vi "three_button.vi"(7 "callee":refnum<vi>, 8 "error in (no error)":errorcluster, 11 "configuration":T2={"dialog_text"="", "boolean_text_1"="", "boolean_text_2"="", "boolean_text_3"="", "inner_color"=16711680, "outer_color"=6618880, "wait_s"=nan, "error_status"=FALSE, "error_source"="", "error_details"="", "string []"=[], "custom_entry"=FALSE}) -> (0 "error out":errorcluster, 3 "dialog_selection":T1)   [LabVIEW 2015, in "lv-dialog-interfaces.lvlib"]
uses:
  lv-dialog-interfaces.lvlib
  lv-dialog/api/v1/public/_controls/configuration.ctl
  lv-dialog/api/v1/public/_controls/dialog_selection.ctl
  _controls/dialog_type.ctl
  _controls/hmi_references.ctl
  <vilib>/event_ctls.llb/eventvkey.ctl
  lv-dialog/api/v1/v1.lvlib
panel:
  out "dialog":string
  in  "button_1":bool
  in  "button_2":bool
  in  "button_3":bool
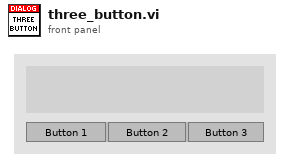
[diagram p1: front panel]
types:
  T1 = typedef "lv-dialog.lvlib/v1.lvlib/dialog_selection.ctl" = enum16{"null", "panel_closed", "button_1", "button_2", "button_3", "cancelled"}
  T2 = typedef "lv-dialog.lvlib/v1.lvlib/configuration.ctl" = cluster{"dialog_text":string, "boolean_text_1":string, "boolean_text_2":string, "boolean_text_3":string, "inner_color":u32, "outer_color":u32, "wait_s":dbl, "error_status":bool, "error_source":string, "error_details":string, "string []":string[], "custom_entry":bool}
  T3 = typedef "lv-dialog-interfaces.lvlib/dialog_type.ctl" = enum16{"null", "one_button", "two_button", "three_button", "confirmation", "busy_wait", "error", "busy_wait_embed", "combo_box", "data_entry_string", "data_entry_numeric"}
  T4 = typedef "lv-dialog-interfaces.lvlib/hmi_references.ctl" = cluster{"vi_reference":refnum<vi>, "caller":refnum<vi>, "dialog":refnum<vi>, "button_1":refnum<vi>, "button_2":refnum<vi>, "button_3":refnum<vi>, "busy":refnum<vi>, "error_glyph":refnum<vi>, "error_source":refnum<vi>, "error_text":refnum<vi>, "combo_box":refnum<vi>}
  T5 = typedef "eventvkey.ctl" = enum16{"ASCII", "Enter", "Return", "Shift", "Ctrl", "Alt", "Cmd", "Opt", "Caps", "NumLock", "Clear", "Break", "Up", "Down", "Left", "Right", "Insert", "Delete", "Home", "End", "PageUp", "PageDown", "Escape", "Help", "Pause", "ScrollLock", "F1", "F2", "F3", "F4", "F5", "F6", "F7", "F8", "F9", "F10", "F11", "F12", "F13", "F14", "F15", "F16", "F17", "F18", "F19", "F20", "F21", "F22", "F23", "F24", "Play", "VolumeUp", "VolumeDown", "Mute", "Two Byte Char"}
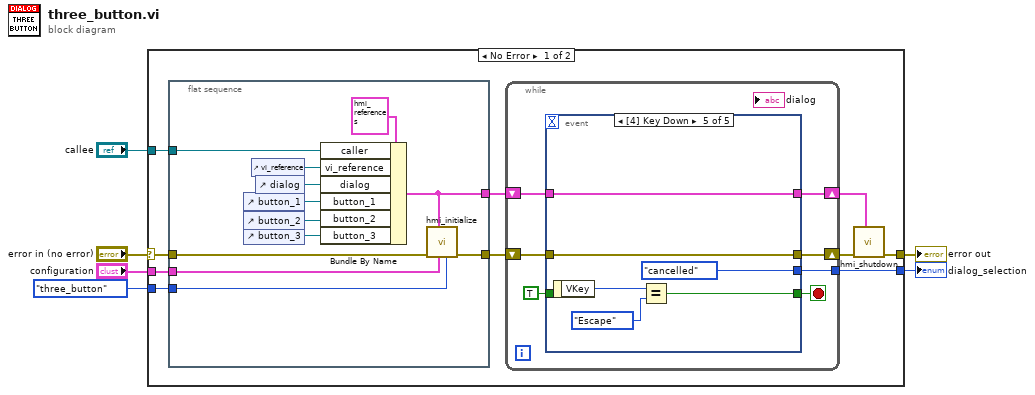
[diagram p0: block diagram]
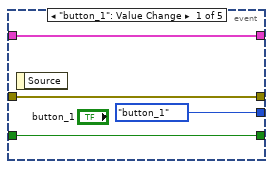
[diagram p2: hidden frame]
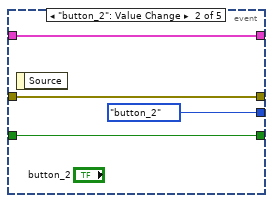
[diagram p3: hidden frame]
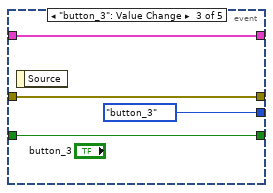
[diagram p4: hidden frame]
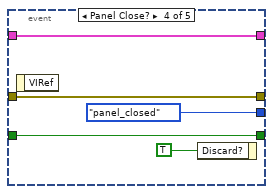
[diagram p5: hidden frame]
diagram:
  n1 = case shown="No Error" "error in (no error)" {
    selector: "error in (no error)" -> [w16 w59]
    tunnel: "configuration" -> [w15 _]
    tunnel: dialog_type."three_button" ("dialog_type") -> [w14 _]
    tunnel: [w12 _] -> w3
    tunnel: "callee" -> [w11 _]
    tunnel: [w8 w59] -> w1
    frame No Error {
      n2 = flat-sequence {
        tunnel: w16 -> [w19]
        tunnel: w15 -> [w24]
        tunnel: w14 -> [w23]
        tunnel: [w22] -> w13
        tunnel: w11 -> [w18]
        tunnel: [w17] -> w10
        frame #0 {
          n3 = control-ref of="button_1"() -> (w26:refnum<vi>)
          n4 = control-ref of="button_2"() -> (w21:refnum<vi>)
          n5 = control-ref of="button_3"() -> (w20:refnum<vi>)
          n6 = control-ref of="vi_reference"() -> (w28:refnum<vi>)
          n7 = control-ref of="dialog"() -> (w27:refnum<vi>)
          n8 = Bundle By Name(cluster=T4 {"vi_reference"=refnum, "caller"=refnum, "dialog"=refnum, "button_1"=refnum, "button_2"=refnum, "button_3"=refnum, "busy"=refnum, "error_glyph"=refnum, "error_source"=refnum, "error_text"=refnum, "combo_box"=refnum}, "caller"=w18, "vi_reference"=w28, "dialog"=w27, "button_1"=w26, "button_2"=w21, "button_3"=w20) -> (w17:T4)
          n9 = call "hmi_initialize.vi"("dialog_type"=w23, "configuration"=w24, "references"=w17, "error in (no error)"=w19) -> ("error out"=w22:errorcluster)  [unwired: 7 in]
        }
      }
      n10 = while {
        tunnel: [w34] -> w12
        shift-right: [w32] -> w9
        shift-left: w13 -> [w35]
        shift-right: [w31] -> w7
        shift-left: w10 -> [w33]
        stop <- w29 stop-if-true
        n11 = event shown="[4] Key Down" {
          selector: _ -> [_ _ _ _ _]
          dyn-events: _ -> [_ _ _ _ _]
          timeout: _ -> [_ _ _ _ _]
          tunnel: w35 -> [w39 w43 w47 w51 w58]
          tunnel: [w39 w43 w47 w51 w58] -> w32
          tunnel: [dialog_selection."button_1" ("dialog_selection") dialog_selection."button_2" ("dialog_selection") dialog_selection."button_3" ("dialog_selection") dialog_selection."panel_closed" ("dialog_selection") dialog_selection."cancelled" ("dialog_selection")] -> w34
          tunnel: w33 -> [w37 w41 w45 w49 w56]
          tunnel: [w37 w41 w45 w49 w56] -> w31
          tunnel: [w36 w40 w44 w48 w53] -> w29
          tunnel: TRUE -> [w36 w40 w44 w48 _]
          event "button_1": Value Change {
            n12 = event-data() -> ()  [unwired: 1 in, 1 out]
          }
          event "button_2": Value Change {
            n13 = event-data() -> ()  [unwired: 1 in, 1 out]
          }
          event "button_3": Value Change {
            n14 = event-data() -> ()  [unwired: 1 in, 1 out]
          }
          event Panel Close? {
            n15 = event-data() -> ()  [unwired: 1 in, 1 out]
            n16 = event-data("Discard?"=TRUE) -> ()  [unwired: 1 in, 1 out]
          }
          event Key Down {
            n17 = event-data() -> ("VKey"=w55:T5)  [unwired: 1 in]
            n18 = Equal?(x=w55, y=eventvkey."Escape" ("VKey")) -> (x = y?=w53:bool)
          }
        }
      }
      n19 = call "hmi_shutdown.vi"("references"=w7, "error in (no error)"=w9) -> ("error out"=w8:errorcluster)  [unwired: 9 in]
    }
    frame Error {
    }
  }
  "error out" <- w1
  "dialog_selection" <- w3
